vi "Set DC Current.vi"(0 "Address":string="24", 1 "Current":dbl format="%.3e") -> ()   [LabVIEW 2012]
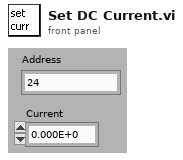
[diagram p1: front panel]
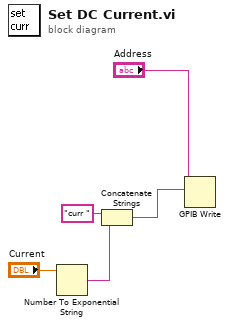
[diagram p0: block diagram]
diagram:
  n1 = Number To Exponential String(number="Current") -> (E-format string=w2:string)  [unwired: 3 in]
  n2 = Concatenate Strings("curr " ("string"), w2) -> (w1:string)
  n3 = GPIB Write(0:"Address", 1:w1) -> ()  [unwired: 3 in, 2 out]
